vi "Selector Status.vi"(8 "error in (no error)":errorcluster, 11 "VISA resource name":refnum<visa-resource-name>) -> (0 "error out":errorcluster, 2 "Selector Option":string, 3 "VISA resource name out":refnum<visa-resource-name>)   [LabVIEW 2015, in "Keysight U1252.lvlib"]
uses:
  <instrlib>/Keysight U1252/Keysight U1252.lvlib
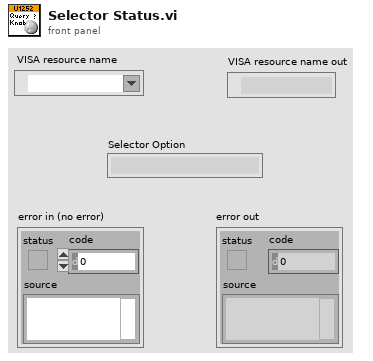
[diagram p1: front panel]
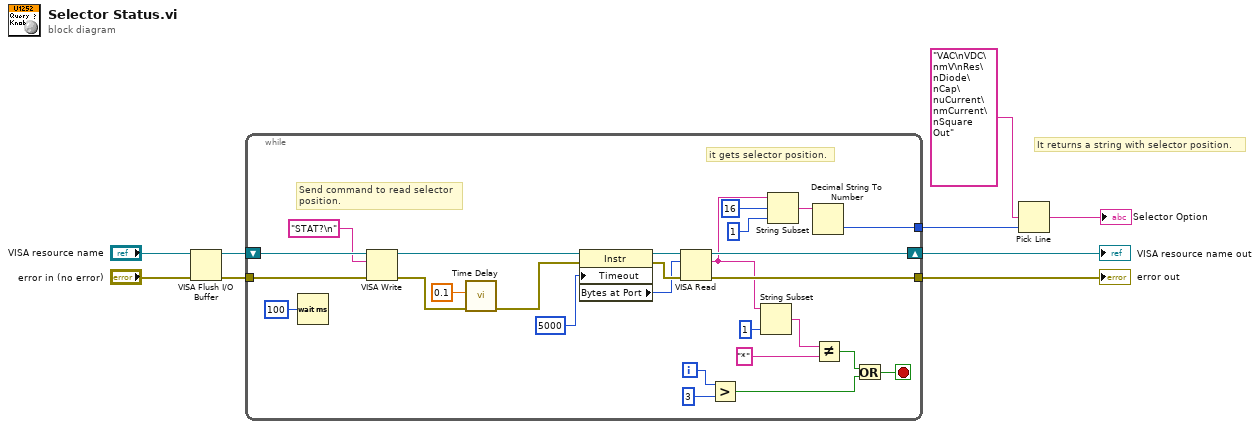
[diagram p0: block diagram]
diagram:
  # "It returns a string with selector position."
  n1 = VISA Flush I/O Buffer(VISA resource name="VISA resource name", error in (no error)="error in (no error)") -> (VISA resource name out=w4:refnum<visa-resource-name>, error out=w5:errorcluster)  [unwired: 1 in]
  n2 = while {
    shift-right: [w35] -> w8
    shift-left: w4 -> [w36]
    tunnel: w5 -> [w27]
    tunnel: [w24] -> w9
    tunnel: [w10] -> w3
    i -> [w29]
    stop <- w16 stop-if-true
    # "it gets selector position."
    # "Send command to read selector\nposition."
    n3 = Wait (ms)(milliseconds to wait=u32 100) -> ()  [unwired: 1 out]
    n4 = VISA Write(VISA resource name=w36, write buffer="STAT?\n", error in (no error)=w27) -> (VISA resource name out=w33:refnum<visa-resource-name>, error out=w19:errorcluster)  [unwired: 1 out]
    n5 = call "Time Delay"("error in (no error)"=w19, "Delay Time (s)"=0.1) -> ("error out"=w18:errorcluster)  [unwired: 9 in]
    n6 = property class="Instr"(reference=w33, error in=w18, "Timeout"=u32 5000 ("General Settings:Timeout Value")) -> (reference out=w31:refnum<visa-resource-name>, error out=w30:errorcluster, "Bytes at Port"=w21:u32)
    n7 = VISA Read(VISA resource name=w31, byte count=w21, error in (no error)=w30) -> (VISA resource name out=w35:refnum<visa-resource-name>, read buffer=w14:string, error out=w24:errorcluster)  [unwired: 1 out]
    n8 = Greater?(x=w29, y=3) -> (0:w15:bool)
    n9 = String Subset(string=w14, length (rest)=1 ("length (rest)")) -> (substring=w22:string)  [unwired: 1 in]
    n10 = String Subset(string=w14, offset (0)=16, length (rest)=1 ("length (rest)")) -> (substring=w11:string)
    n11 = Decimal String To Number(string=w11) -> (number=w10:i32)  [unwired: 2 in, 1 out]
    n12 = Not Equal?(x=w22, y="*") -> (x != y?=w17:bool)
    n13 = Or(x=w17, y=w15) -> (x .or. y?=w16:bool)
  }
  "error out" <- w9
  "VISA resource name out" <- w8
  n14 = Pick Line(multi-line string="VAC\nVDC\nmV\nRes\nDiode\nCap\nuCurrent\nmCurrent\nSquare Out", line index=w3) -> (output string=→"Selector Option":string)  [unwired: 1 in]
